vi "Serial_getc.vi"(8 "error in (no error)":errorcluster, 11 "Serial in":refnum<class "Serial.lvclass">) -> (0 "error out":errorcluster, 2 "char":i32, 3 "Serial out":refnum<class "Serial.lvclass">)   [LabVIEW 2011, in "mbed_LVLibrary.lvlib" / "Serial.lvclass"]
doc: "Reads a character from the serial port on mbed"
uses:
  Serial.lvclass
  Serial.lvclass/Serial.ctl
  Transport Mechanisms/mbed/mbed.lvclass
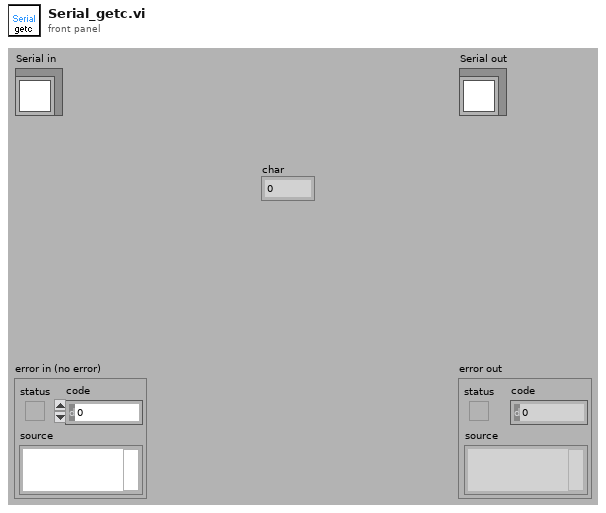
[diagram p1: front panel]
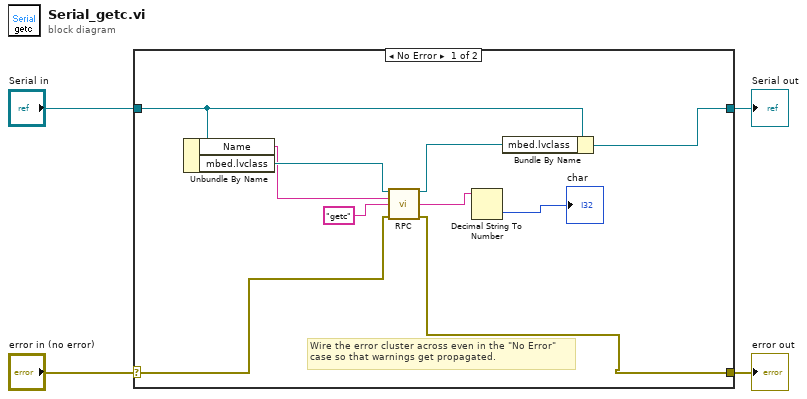
[diagram p0: block diagram]
diagram:
  n1 = case shown="No Error" "error in (no error)" {
    selector: "error in (no error)" -> [w6 w16]
    tunnel: [w5 w16] -> w3
    tunnel: [w8 w15] -> w1
    tunnel: "Serial in" -> [w9 w15]
    frame No Error {
      # "Wire the error cluster across even in the \"No Error\"\ncase so that warnings get propagated."
      n2 = Unbundle By Name(w9) -> ("Name"=w13:string, "mbed.lvclass"=w14:refnum<class "mbed.lvclass">)
      n3 = call-dynamic "RPC.vi"("mbed in"=w14, "Name"=w13, "method"="getc", "error in (no error)"=w6) -> ("mbed out"=w7:refnum<class "mbed.lvclass">, "RPC Result"=w11:string, "error out"=w5:errorcluster)  [unwired: 9 in]
      n4 = Decimal String To Number(string=w11) -> (number=→"char":i32)  [unwired: 2 in, 1 out]
      n5 = Bundle By Name(cluster=w9, "mbed.lvclass"=w7) -> (w8:refnum<class "Serial.lvclass">)
    }
    frame Error {
    }
  }
  "error out" <- w3
  "Serial out" <- w1
